vi "X Coil Current to Magnetic field (SubVI).vi"(11 "Current X":dbl) -> (3 "Magnetic field X [µT]":string)   [LabVIEW 2018]
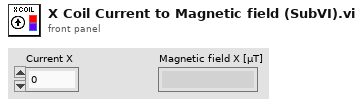
[diagram p1: front panel]
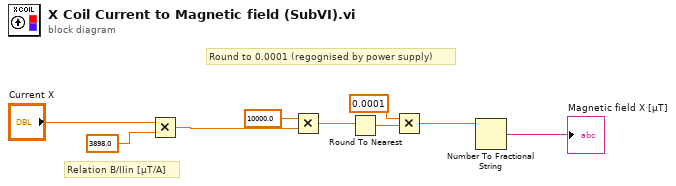
[diagram p0: block diagram]
diagram:
  # "Round to 0.0001 (regognised by power supply)"
  # "Relation B/IIin [µT/A]"
  n1 = Multiply(x="Current X", y=3898.0) -> (x*y=w2:dbl)
  n2 = Multiply(x=10000.0, y=w2) -> (x*y=w5:dbl)
  n3 = Round To Nearest(number=w5) -> (nearest integer value=w4:dbl)
  n4 = Multiply(x=0.0001, y=w4) -> (x*y=w1:dbl)
  n5 = Number To Fractional String(number=w1) -> (F-format string=→"Magnetic field X [µT]":string)  [unwired: 3 in]
